vi "Begin.vi"() -> ()   [LabVIEW 2017]
doc: "Called before other user functions, this VI is expected to open initial I/O refnums, load in file data, and do all program initialization. Notice that the <B>error out</B> terminal is simply used for data flow. Wiring it to other structures or subVIs ensures that this VI runs first."
uses:
  TankDrivePreseason/RightMotors.ctl
  TankDrivePreseason/LeftMotors.ctl
  <vilib>/Rock Robotics/WPI/ThirdParty/Phoenix-LabVIEW/Pigeon IMU/CTRE_PigeonIMU_Open_TalonSRX.vi
panel:
  in  "error in":errorcluster
  out "error out":errorcluster
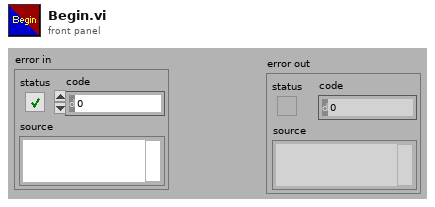
[diagram p1: front panel]
types:
  T1 = typedef "LeftMotors.ctl" = enum16{"LMotor 1", "LMotor 2", "LMotor 3"}
  T2 = typedef "RightMotors.ctl" = enum16{"RMotor 1", "RMotor 2", "RMotor 3"}
  T3 = typedef "WPI_MotorControlDeviceRef.ctl" = cluster{"DeviceStatus":errorcluster, "Type":T4, "PWM":cluster{"PWM Channel":T5, "DeadBand":T6}, "CAN":cluster{"Device Number":u8, "SetOutput VI Ref":variant, "GetOutput VI Ref":variant, "Enable VI Ref":variant, "Disable VI Ref":variant, "Data":variant}, "Invert":bool, "DIO PWM":cluster{"PWM \"Enable\" Channel":T5, "DIOChannel":T7, "PWM Rate":dbl}}
  T4 = typedef "WPI_MotorControlType.ctl" = enum16{"PWM", "CAN", "DIO PWM"}
  T5 = typedef "FPGA_DIOPWMChannel.ctl" = enum8{"PWM 0", "PWM 1", "PWM 2", "PWM 3", "PWM 4", "PWM 5", "PWM 6", "PWM 7", "PWM 8", "PWM 9", "PWM MXP 0", "PWM MXP 1", "PWM MXP 2", "PWM MXP 3", "PWM MXP 4", "PWM MXP 5", "PWM MXP 6", "PWM MXP 7", "PWM MXP 8", "PWM MXP 9", "Invalid"}
  T6 = typedef "WPI_PWMDeadband.ctl" = cluster{"Name":string, "maxPositivePwm":i32, "minPositivePwm":i32, "centerPwm":i32, "maxNegativePwm":i32, "minNegativePwm":i32, "angularRange":u16}
  T7 = typedef "FPGA_DIOChannel.ctl" = enum8{"DIO 0", "DIO 1", "DIO 2", "DIO 3", "DIO 4", "DIO 5", "DIO 6", "DIO 7", "DIO 8", "DIO 9", "DIO MXP 0", "DIO MXP 1", "DIO MXP 2", "DIO MXP 3", "DIO MXP 4", "DIO MXP 5", "DIO MXP 6", "DIO MXP 7", "DIO MXP 8", "DIO MXP 9", "DIO MXP 10", "DIO MXP 11", "DIO MXP 12", "DIO MXP 13", "DIO MXP 14", "DIO MXP 15", "SPI Port CS1", "SPI Port CS2", "SPI Port CS3", "SPI Port MISO", "SPI Port MOSI", "Invalid"}
  T8 = typedef "CTRE_PigeonIMU_DeviceRef.ctl" = cluster{"DeviceStatus":errorcluster, "Device Number":u8, "Type":T9, "Device ID":u32, "Handle":u64, "UsageFrame":u32, "Library Path":path}
  T9 = typedef "CTRE_PigeonIMU_ConnectionType.ctl" = u32
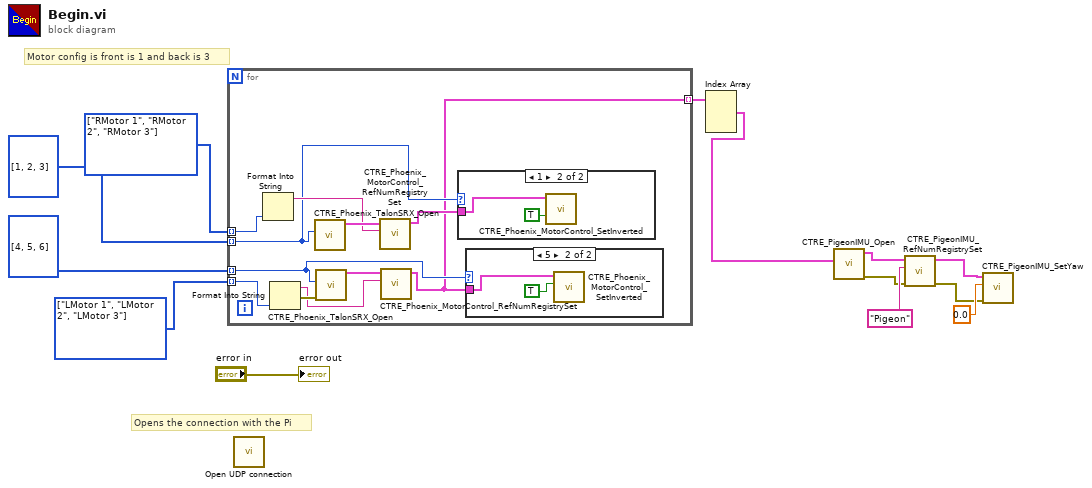
[diagram p0: block diagram]
diagram:
  w12 = T1[] [enum."LMotor 1", enum."LMotor 2", enum."LMotor 3"] items=["LMotor 1", "LMotor 2", "LMotor 3"]
  w11 = T2[] [enum."RMotor 1", enum."RMotor 2", enum."RMotor 3"] items=["RMotor 1", "RMotor 2", "RMotor 3"]
  # "Opens the connection with the Pi"
  # "Motor config is front is 1 and back is 3"
  n1 = for {
    tunnel: w12 -> [w20] mode=indexing
    tunnel: w11 -> [w23] mode=indexing
    tunnel: i32[] [4, 5, 6] -> [w16] mode=indexing
    tunnel: i32[] [1, 2, 3] -> [w17] mode=indexing
    tunnel: [w14] -> w4 mode=indexing
    n2 = Format Into String(w23) -> (resulting string=w22:string)  [unwired: 3 in, 1 out]
    n3 = Format Into String(w20) -> (resulting string=w19:string, error out=w21:errorcluster)  [unwired: 3 in]
    n4 = call <vilib>:"CTRE_Phoenix_TalonSRX_Open.vi"("Device Number"=w17) -> ("CAN Talon SRX Ref"=w24:T3)  [unwired: 9 in, 1 out]
    n5 = call <vilib>:"CTRE_Phoenix_TalonSRX_Open.vi"("error in"=w21, "Device Number"=w16) -> ("CAN Talon SRX Ref"=w18:T3)  [unwired: 8 in, 1 out]
    n6 = call <vilib>:"CTRE_Phoenix_MotorControl_RefNumRegistrySet.vi"("refnum name"=w22, "PhoenixMotorControlDevRef"=w24) -> ("PhoenixMotorControlDevRef"=w15:T3)  [unwired: 8 in, 1 out]
    n7 = call <vilib>:"CTRE_Phoenix_MotorControl_RefNumRegistrySet.vi"("refnum name"=w19, "PhoenixMotorControlDevRef"=w18) -> ("PhoenixMotorControlDevRef"=w14:T3)  [unwired: 8 in, 1 out]
    n8 = case shown="1" w17 {
      tunnel: w15 -> [_ w28]
      frame Default {
      }
      frame 1 {
        n9 = call <vilib>:"CTRE_Phoenix_MotorControl_SetInverted.vi"("Invert?"=TRUE, "PhoenixMotorControlDevRef"=w28) -> ()  [unwired: 8 in, 2 out]
      }
    }
    n10 = case shown="5" w16 {
      tunnel: w14 -> [_ w26]
      frame Default {
      }
      frame 5 {
        n11 = call <vilib>:"CTRE_Phoenix_MotorControl_SetInverted.vi"("Invert?"=TRUE, "PhoenixMotorControlDevRef"=w26) -> ()  [unwired: 8 in, 2 out]
      }
    }
  }
  n12 = call "Open UDP connection.vi"() -> ()  [unwired: 12 in]
  n13 = Index Array(array=w4) -> (element #1=w3:T3)  [unwired: 3 in, 2 out]
  n14 = call-poly <vilib>:"CTRE_PigeonIMU_Open.vi"("CAN Talon SRX Ref"=w3) -> ("error out"=w1:errorcluster, "PigeonIMUDevRef"=w8:T8)  [unwired: 9 in]
  n15 = call <vilib>:"CTRE_PigeonIMU_RefNumRegistrySet.vi"("error in (no error)"=w1, "refnum name"="Pigeon", "PigeonIMUDevRef"=w8) -> ("error out"=w2:errorcluster, "PigeonIMUDevRef"=w6:T8)  [unwired: 7 in]
  n16 = call <vilib>:"CTRE_PigeonIMU_SetYaw.vi"("error in (no error)"=w2, "Value"=0.0, "PigeonIMUDevRef"=w6) -> ()  [unwired: 7 in, 2 out]
  "error out" <- "error in"
